vi "2018新生赛半成品.vi"() -> ()   [LabVIEW 2013]
doc: "本范例根据用户指示，对串口执行读写操作。范例运行时可按下“写入”或“读取”按钮，以及修改“读数”。\n\n设置的串口参数必须匹配连接仪器或设备的参数。本范例中，“读数”参数可指定串口读取的字节数。如端口字节超过指定的字节数，超出部分将不会被读取。如端口字节数少于指定的字节数，将返回超时错误。\n\n本范例可扩展流控制选项以包括XON和XOFF，从而允许用户选择控制字符。同时，用户可启用或禁用中止符。部分设备需要通过终止符确定命令字符串的结束位置。部分设备将发送终止符以说明待读取数据的末端。本范例演示了缓冲区中检测到终止符时，结束“读取”操作或添加终止符至“写入”数据末端的方法。"
uses:
  E:/National Instruments/LabVIEW 2013/examples/Instrument IO/Serial/support/Serial - Settings.ctl
  <vilib>/Instr/_visa.llb/VISA Configure Serial Port (Instr).vi
panel:
  out "L":u8
  out "R":u8
  out "D":u8
  out "R":i16(slide) scale=-255.0..255.0
  out "L":i16(slide) scale=-255.0..255.0
  out "DY":u8
  out "DX":u8
  out "TY":u8
  out "TX":u8
  out "HY":u8
  out "HX":u8
  in  "读取":bool
  out "响应":string
  in  "读数":u32=1000
  in  "VISA资源名称 读取":refnum<visa-resource-name>="COM1"
  in  "串口设置 读取":T1={"波特率"=9600, "数据比特"=8, "奇偶"=enum."None", "停止位"=10, "流控制"=0} {"流控制" items=["无"=0, "XON/XOFF"=1, "RTS/CTS"=2, "DTR/DSR"=4]; "停止位" items=["1.0"=10, "1.5"=15, "2.0"=20]; "数据比特" min=5 max=8 step=1; "波特率" items=["75"=75, "110"=110, "134"=134, "150"=150, "300"=300, "600"=600, "1200"=1200, "1800"=1800, "2400"=2400, "4800"=4800, "7200"=7200, "9600"=9600, "14400"=14400, "19200"=19200, "28800"=28800, "38400"=38400, "56000"=56000, "57600"=57600, "115200"=115200, "128000"=128000, "230400"=230400]}
  in  "终止符时结束读取？":bool=TRUE
  in  "终止符":u8=10 format="%.0x"
  in  "终止符时结束写入？":bool=TRUE
  in  "停止":bool
  out "命令":string="*IDN?"
  in  "写入":bool
  in  "串口设置 写入":T1={"波特率"=9600, "数据比特"=8, "奇偶"=enum."None", "停止位"=10, "流控制"=0} {"流控制" items=["无"=0, "XON/XOFF"=1, "RTS/CTS"=2, "DTR/DSR"=4]; "停止位" items=["1.0"=10, "1.5"=15, "2.0"=20]; "数据比特" min=5 max=8 step=1; "波特率" items=["75"=75, "110"=110, "134"=134, "150"=150, "300"=300, "600"=600, "1200"=1200, "1800"=1800, "2400"=2400, "4800"=4800, "7200"=7200, "9600"=9600, "14400"=14400, "19200"=19200, "28800"=28800, "38400"=38400, "56000"=56000, "57600"=57600, "115200"=115200, "128000"=128000, "230400"=230400]}
  in  "VISA资源名称 写入":refnum<visa-resource-name>="COM1"
  # "概述：演示在循环中使用VISA函数连续写入命令至串口仪器或从串口仪器读取响应。\n要求：NI-VISA驱动程序\n操作步骤：\n1. 运行VI。\n2. 指定命令并单击写入按钮。\n3. 单击读取按钮读取响应。\n4. 单击停止按钮停止VI。"
  # "0xA相当于'\\n'字符，为换行符。"
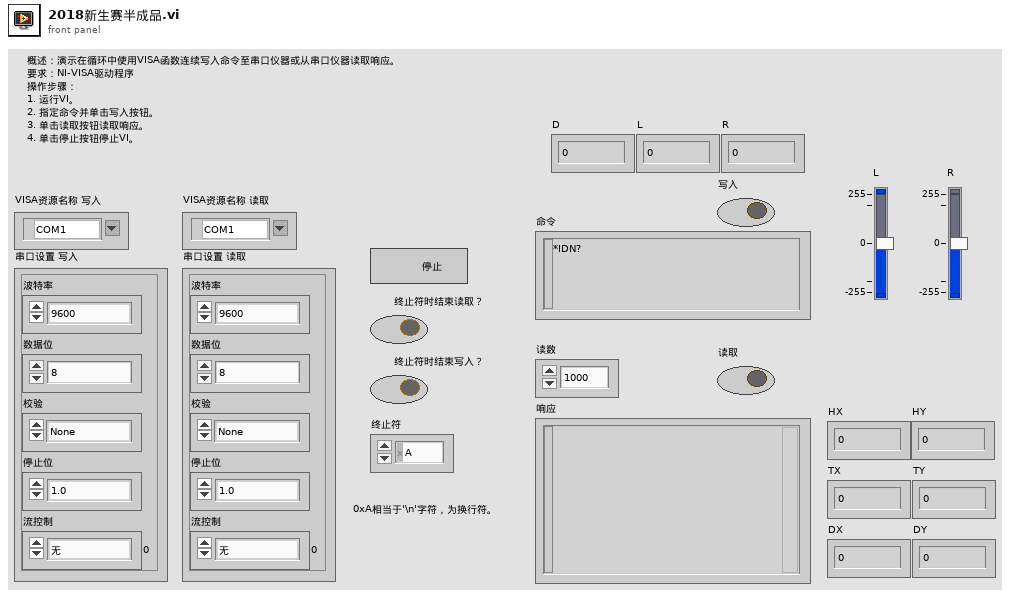
[diagram p1: front panel]
types:
  T1 = typedef "Serial - Settings.ctl" = cluster{"波特率":u32, "数据比特":u16, "奇偶":enum16{"None", "Odd", "Even", "Mark", "Space"}, "停止位":u16, "流控制":u16}
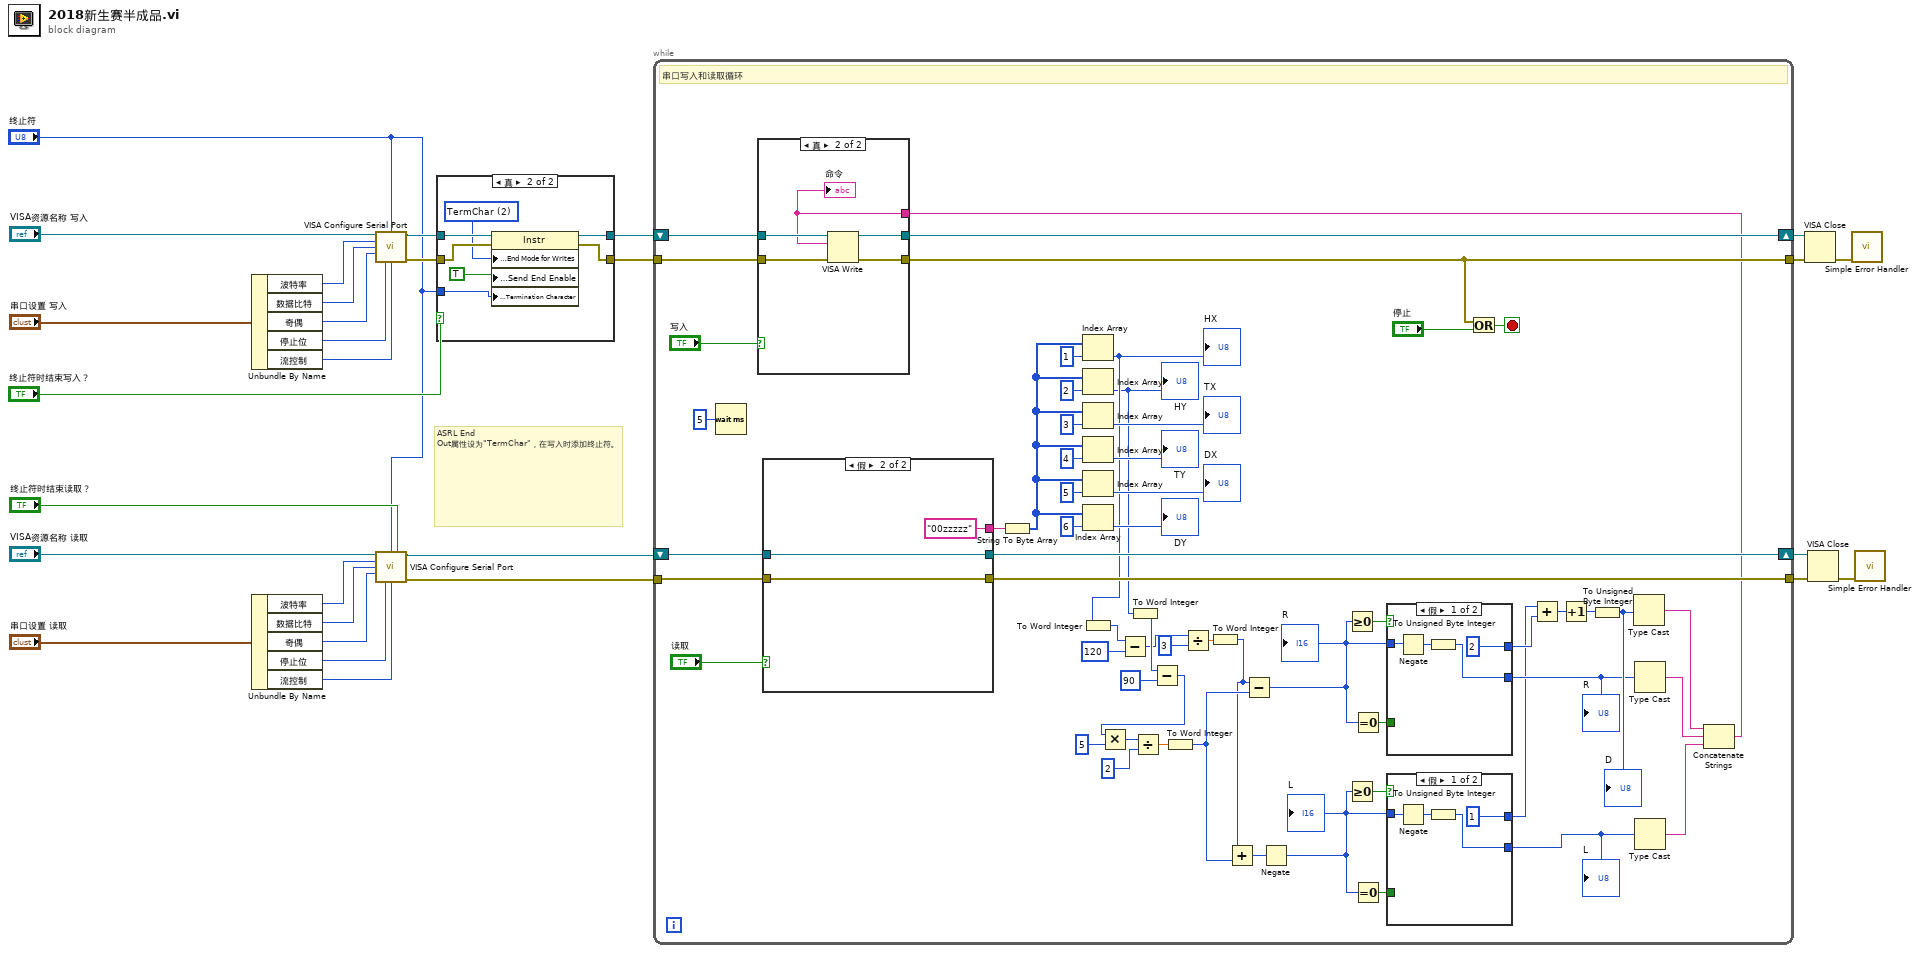
[diagram p0: block diagram]
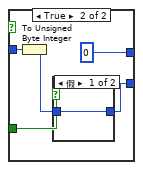
[diagram p3: hidden frame]
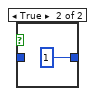
[diagram p4: hidden frame]
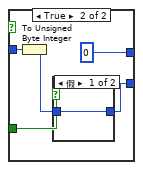
[diagram p5: hidden frame]
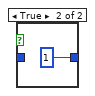
[diagram p6: hidden frame]
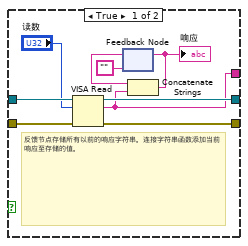
[diagram p7: hidden frame]
diagram:
  # "ASRL End Out属性设为\"TermChar\"，在写入时添加终止符。"
  n1 = Unbundle By Name("串口设置 写入") -> ("波特率"=w25:u32, "数据比特"=w26:u16, "奇偶"=w27:enum16{"None", "Odd", "Even", "Mark", "Space"}, "停止位"=w28:u16, "流控制"=w21:u16)
  n2 = Unbundle By Name("串口设置 读取") -> ("波特率"=w13:u32, "数据比特"=w14:u16, "奇偶"=w15:enum16{"None", "Odd", "Even", "Mark", "Space"}, "停止位"=w16:u16, "流控制"=w9:u16)
  n3 = call-poly "VISA Configure Serial Port"("VISA resource name"="VISA资源名称 写入", "termination char\n(0xA = '\\n' = LF)"="终止符", "baud rate (9600)"=w25, "data bits (8)"=w26, "parity (0:none)"=w27, "stop bits (10: 1 bit)"=w28, "flow control (0:none)"=w21) -> ("VISA resource name out"=w7:refnum<visa-resource-name>, "error out"=w6:errorcluster)  [unwired: 3 in, 4 out]
  n4 = call-poly "VISA Configure Serial Port"("VISA resource name"="VISA资源名称 读取", "termination char\n(0xA = '\\n' = LF)"="终止符", "Enable Termination\nChar (T)"="终止符时结束读取？", "baud rate (9600)"=w13, "data bits (8)"=w14, "parity (0:none)"=w15, "stop bits (10: 1 bit)"=w16, "flow control (0:none)"=w9) -> ("VISA resource name out"=w3:refnum<visa-resource-name>, "error out"=w2:errorcluster)  [unwired: 2 in, 4 out]
  n5 = case shown="真" "终止符时结束写入？" {
    tunnel: w7 -> [w30 w38]
    tunnel: w6 -> [w31 w37]
    tunnel: [w30 w36] -> w19
    tunnel: [w31 w35] -> w20
    tunnel: "终止符" -> [_ w33]
    frame False {
    }
    frame True {
      w34 = u16 2 items=["None", "LastBit", "TermChar", "Break"] ("Serial Settings:Serial End Mode for Writes")
      n6 = property class="Instr"(reference=w38, error in=w37, "Serial Settings:End Mode for Writes"=w34, "Message Based Settings:Send End Enable"=TRUE, "Message Based Settings:Termination Character"=w33) -> (reference out=w36:refnum<visa-resource-name>, error out=w35:errorcluster)
    }
  }
  n7 = while {
    shift-right: [w87] -> w22
    shift-left: w19 -> [w97]
    tunnel: w20 -> [w96]
    tunnel: w2 -> [w88]
    shift-right: [w90] -> w8
    shift-left: w3 -> [w89]
    tunnel: [w86] -> w5
    tunnel: [w85] -> w4
    stop <- w94 stop-if-true
    # "串口写入和读取循环"
    n8 = Wait (ms)(milliseconds to wait=u32 5) -> ()  [unwired: 1 out]
    n9 = case shown="假" "读取" {
      tunnel: [w126 w131] -> w90
      tunnel: w89 -> [w128 w131]
      tunnel: [w124 w130] -> w85
      tunnel: w88 -> [w127 w130]
      tunnel: [w120 "00zzzzz" ("read buffer")] -> w81
      frame True {
        # "反馈节点存储所有以前的响应字符串。连接字符串函数添加当前响应至存储的值。"
        n10 = VISA Read(VISA resource name=w128, byte count="读数", error in (no error)=w127) -> (VISA resource name out=w126:refnum<visa-resource-name>, read buffer=w120:string, error out=w124:errorcluster)  [unwired: 1 out]
        n11 = feedback #1("") -> (w123:string)
        n12 = Concatenate Strings(w123, w120) -> (w121:string)
        "响应" <- w121
        n13 = feedback-in #1(w121) -> ()
      }
      frame False {
      }
    }
    n14 = String To Byte Array(string=w81) -> (unsigned byte array=w80:u8[])
    n15 = Index Array(array=w80, index=1 ("索引")) -> (element=w52:u8)
    "HX" <- w52
    n16 = Index Array(array=w80, index=2 ("索引")) -> (element=w50:u8)
    "HY" <- w50
    n17 = Index Array(array=w80, index=3 ("索引")) -> (element=→"TX":u8)
    n18 = Index Array(array=w80, index=4 ("索引")) -> (element=→"TY":u8)
    n19 = Index Array(array=w80, index=5 ("索引")) -> (element=→"DX":u8)
    n20 = Index Array(array=w80, index=6 ("索引")) -> (element=→"DY":u8)
    n21 = To Word Integer(number=w52) -> (16bit integer=w51:i16)
    n22 = Subtract(x=w51, y=i16 120) -> (x-y=w40:i16)
    n23 = To Word Integer(number=w50) -> (16bit integer=w49:i16)
    n24 = Subtract(x=w49, y=i16 90) -> (x-y=w47:i16)
    n25 = Multiply(x=w47, y=i16 5) -> (x*y=w48:i16)
    n26 = Divide(x=w48, y=i16 2) -> (x/y=w44:dbl)
    n27 = To Word Integer(number=w44) -> (16bit integer=w43:i16)
    n28 = Divide(x=w40, y=i16 3) -> (x/y=w42:dbl)
    n29 = To Word Integer(number=w42) -> (16bit integer=w41:i16)
    n30 = Add(x=w41, y=w43) -> (x+y=w55:i16)
    n31 = Subtract(x=w41, y=w43) -> (x-y=w53:i16)
    "R" <- w53
    n32 = Negate(x=w55) -> (-x=w54:i16)
    "L" <- w54
    n33 = Greater Or Equal To 0?(x=w53) -> (x >= 0?=w63:bool)
    n34 = Greater Or Equal To 0?(x=w54) -> (x >= 0?=w61:bool)
    n35 = Equal To 0?(x=w53) -> (x = 0?=w62:bool)
    n36 = Equal To 0?(x=w54) -> (x = 0?=w60:bool)
    n37 = case shown="假" w63 {
      tunnel: w53 -> [w112 w116]
      tunnel: [w111 w113] -> w65
      tunnel: [2 0] -> w68
      tunnel: w62 -> [_ w115]
      frame False {
        n38 = Negate(x=w112) -> (-x=w109:i16)
        n39 = To Unsigned Byte Integer(number=w109) -> (unsigned 8bit integer=w111:u8)
      }
      frame True {
        n40 = To Unsigned Byte Integer(number=w116) -> (unsigned 8bit integer=w114:u8)
        n41 = case shown="假" w115 {
          tunnel: w114 -> [w118 _]
          tunnel: [w118 u8 1] -> w113
          frame False {
          }
          frame True {
          }
        }
      }
    }
    "R" <- w65
    n42 = case shown="假" w61 {
      tunnel: [w101 w103] -> w58
      tunnel: [1 0] -> w59
      tunnel: w60 -> [_ w105]
      tunnel: w54 -> [w98 w102]
      frame False {
        n43 = Negate(x=w98) -> (-x=w99:i16)
        n44 = To Unsigned Byte Integer(number=w99) -> (unsigned 8bit integer=w101:u8)
      }
      frame True {
        n45 = To Unsigned Byte Integer(number=w102) -> (unsigned 8bit integer=w104:u8)
        n46 = case shown="假" w105 {
          tunnel: w104 -> [w107 _]
          tunnel: [w107 u8 1] -> w103
          frame False {
          }
          frame True {
          }
        }
      }
    }
    "L" <- w58
    n47 = Add(x=w59, y=w68) -> (x+y=w69:i32)
    n48 = Increment(x=w69) -> (x+1=w67:i32)
    n49 = To Unsigned Byte Integer(number=w67) -> (unsigned 8bit integer=w66:u8)
    "D" <- w66
    n50 = Type Cast(x=w66) -> (*(type *) &x=w84:string)  [unwired: 1 in]
    n51 = Type Cast(x=w65) -> (*(type *) &x=w83:string)  [unwired: 1 in]
    n52 = Type Cast(x=w58) -> (*(type *) &x=w82:string)  [unwired: 1 in]
    n53 = Concatenate Strings(w84, w83, w82) -> (w64:string)
    n54 = case shown="真" "写入" {
      tunnel: w97 -> [w133 w138]
      tunnel: w96 -> [w132 w137]
      tunnel: [w133 w136] -> w87
      tunnel: [w132 w135] -> w86
      tunnel: w64 -> [_ w134]
      frame False {
      }
      frame True {
        n55 = VISA Write(VISA resource name=w138, write buffer=w134, error in (no error)=w137) -> (VISA resource name out=w136:refnum<visa-resource-name>, error out=w135:errorcluster)  [unwired: 1 out]
        "命令" <- w134
      }
    }
    n56 = Or(x=w86, y="停止") -> (x .or. y?=w94:bool)
  }
  n57 = VISA Close(VISA resource name=w22, error in (no error)=w5) -> (error out=w23:errorcluster)
  n58 = VISA Close(VISA resource name=w8, error in (no error)=w4) -> (error out=w10:errorcluster)
  n59 = call <vilib>:"Simple Error Handler.vi"("error in (no error)"=w23) -> ()  [unwired: 1 in, 8 out]
  n60 = call <vilib>:"Simple Error Handler.vi"("error in (no error)"=w10) -> ()  [unwired: 1 in, 8 out]
